vi "Get Many Attributes Priv.vi"(0 "Tree Dictionary In":variant, 5 "Unique ID":string, 7 "Attribute Names":string[](array[string]), 11 "error in":errorcluster) -> (4 "Tree Dictionary Out":variant, 6 "Attribute Names":string[](array[string]), 8 "Found?":bool[](array[boolean]), 10 "Attribute Values":variant[](array[variant]), 15 "error out":errorcluster)   [LabVIEW 2020, in "NI_VIAnCFGDataStructure.lvlib" / "Tree.lvclass"]
uses:
  <vilib>/addons/analyzer/VIAnCFGDataStructure/Tree Manager/Tree.lvclass
  <vilib>/addons/analyzer/VIAnCFGDataStructure/Tree Manager/Typedefs/Tree Cluster.ctl
  <vilib>/Utility/error.llb/Error Cluster From Error Code.vi
  <vilib>/ErrorRing/Error Ring.xnode
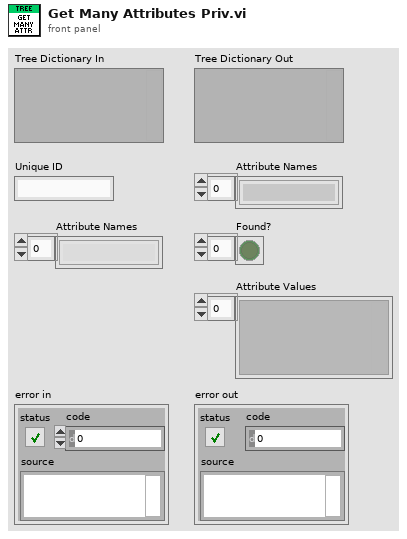
[diagram p1: front panel]
types:
  T1 = typedef "NI_VIAnCFGDataStructure.lvlib/Tree.lvclass/Tree Cluster.ctl" = cluster{"Unique ID":string, "Parent ID":string, "Child IDs":string[], "Name":string, "MetaData":string, "Data IDs":string[]}
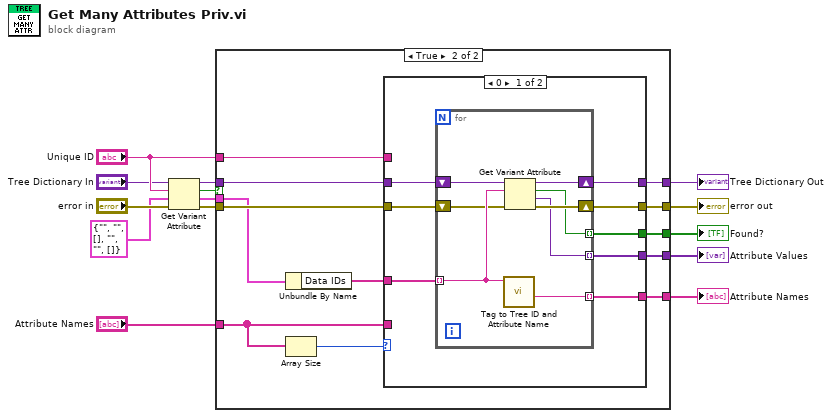
[diagram p0: block diagram]
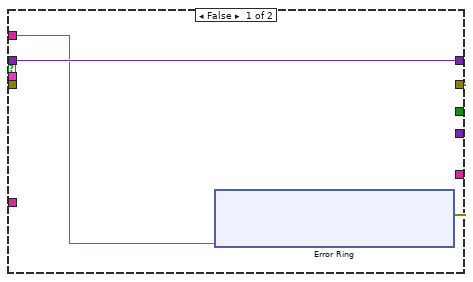
[diagram p2: hidden frame]
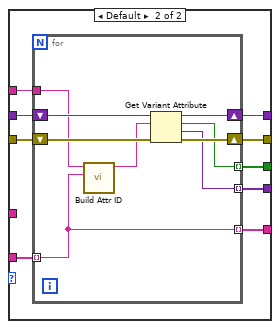
[diagram p3: hidden frame]
diagram:
  n1 = Get Variant Attribute(Variant="Tree Dictionary In", name="Unique ID", default value (empty Variant)=T1 {"Unique ID"="", "Parent ID"="", "Child IDs"=[], "Name"="", "MetaData"="", "Data IDs"=[]} ("Cluster of class private data"), error in="error in") -> (duplicate Variant=w11:variant, found=w12:bool, value=w13:T1, error out=w9:errorcluster)
  n2 = case shown="True" w12 {
    tunnel: [w16 w35] -> w7
    tunnel: [w17 w26] -> w8
    tunnel: w9 -> [_ w36]
    tunnel: w11 -> [w17 w27]
    tunnel: w13 -> [_ w32]
    tunnel: "Unique ID" -> [w15 w25]
    tunnel: [_ w34] -> w2
    tunnel: [_ w33] -> w4
    tunnel: "Attribute Names" -> [_ w30]
    tunnel: [_ w28] -> w1
    frame False {
      n3 = xnode "Error Ring"("parameter 0"=w15) -> ("error out"=w16:errorcluster)
    }
    frame True {
      n4 = Unbundle By Name(w32) -> ("Data IDs"=w31:string[])
      n5 = Array Size(array=w30) -> (size(s)=w29:i32)
      n6 = case shown="0" w29 {
        tunnel: w36 -> [w41 w61]
        tunnel: [w40 w60] -> w35
        tunnel: [w37 w59] -> w34
        tunnel: [w38 w58] -> w33
        tunnel: w31 -> [w43 _]
        tunnel: w30 -> [_ w57]
        tunnel: [w42 w56] -> w28
        tunnel: w27 -> [w44 w55]
        tunnel: [w39 w53] -> w26
        tunnel: w25 -> [_ w54]
        frame 0 {
          n7 = for {
            shift-right: [w51] -> w39
            shift-left: w44 -> [w52]
            tunnel: w43 -> [w50] mode=indexing
            tunnel: [w49] -> w42 mode=indexing
            shift-right: [w47] -> w40
            shift-left: w41 -> [w48]
            tunnel: [w46] -> w38 mode=indexing
            tunnel: [w45] -> w37 mode=indexing
            n8 = call <vilib>:"Tag to Tree ID and Attribute Name.vi"("Tag"=w50) -> ("Attribute Name"=w49:string)  [unwired: 8 in, 2 out]
            n9 = Get Variant Attribute(Variant=w52, name=w50, error in=w48) -> (duplicate Variant=w51:variant, found=w45:bool, value=w46:variant, error out=w47:errorcluster)  [unwired: 1 in]
          }
        }
        frame Default {
          n10 = for {
            tunnel: [w68] -> w59 mode=indexing
            tunnel: [w67] -> w58 mode=indexing
            shift-right: [w69] -> w60
            shift-left: w61 -> [w70]
            shift-right: [w66] -> w53
            shift-left: w55 -> [w65]
            tunnel: w57 -> [w62] mode=indexing
            tunnel: [w62] -> w56 mode=indexing
            tunnel: w54 -> [w64]
            n11 = call <vilib>:"Build Attr ID.vi"("Attr Name"=w62, "Unique ID"=w64) -> ("Attr ID Out"=w63:string)  [unwired: 9 in]
            n12 = Get Variant Attribute(Variant=w65, name=w63, error in=w70) -> (duplicate Variant=w66:variant, found=w68:bool, value=w67:variant, error out=w69:errorcluster)  [unwired: 1 in]
          }
        }
      }
    }
  }
  "Tree Dictionary Out" <- w8
  "error out" <- w7
  "Attribute Values" <- w4
  "Found?" <- w2
  "Attribute Names" <- w1
